vi "Marker Y Axes Values.vi"(0 "VISA resource name":refnum<visa-resource-name>, 5 "error in (no error)":errorcluster) -> (8 "o Marker A Value":dbl format="%^.3e", 9 "Right - Left Diff Curs Value":dbl format="%^.3e", 10 "x Marker A Value":dbl format="%^.3e", 11 "Line Curs Right Value":dbl format="%^.3e", 12 "o - x Diff Marker A Value":dbl format="%^.3e", 13 "Line Curs Left Value":dbl format="%^.3e", 14 "VISA resource name out":refnum<visa-resource-name>, 15 "o Marker B Value":dbl format="%^.3e", 16 "x Marker B Value":dbl format="%^.3e", 17 "o - x Diff Marker B Value":dbl format="%^.3e", 18 "Line Curs Value":dbl format="%^.3e", 19 "error out":errorcluster)   [LabVIEW 2017, in "Agilent 4194.lvlib"]
doc: "This function outputs the markers and cursors data valid for Y axis."
uses:
  ISOMems/Agilent 4194/Agilent 4194.lvlib
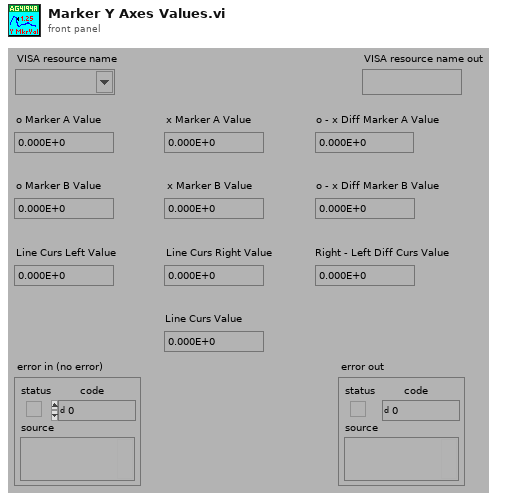
[diagram p1: front panel]
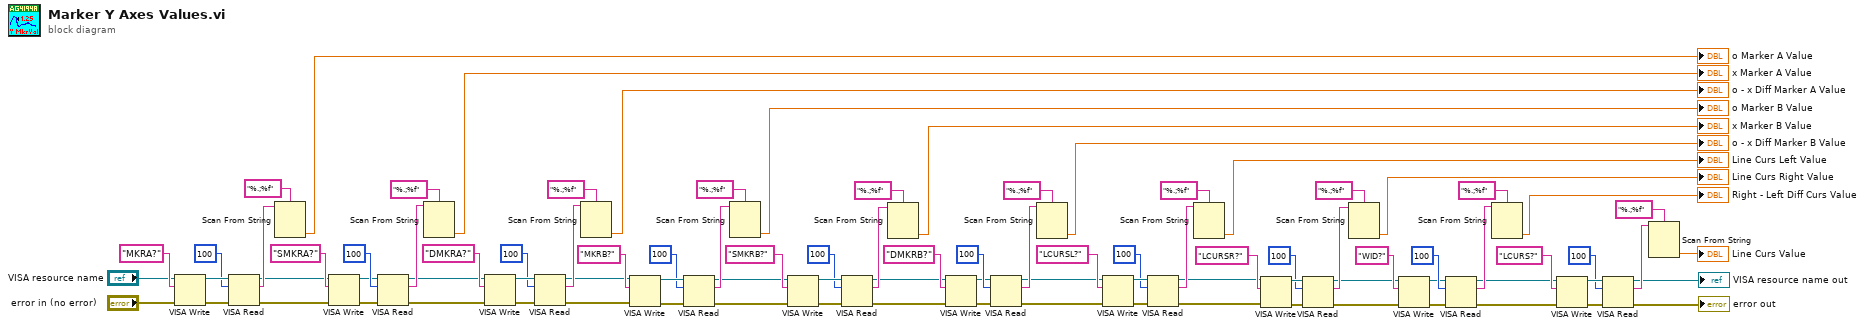
[diagram p0: block diagram]
diagram:
  n1 = VISA Write(VISA resource name="VISA resource name", write buffer="MKRA?" ("write buffer (\"\")"), error in (no error)="error in (no error)") -> (VISA resource name out=w32:refnum<visa-resource-name>, error out=w33:errorcluster)  [unwired: 1 out]
  n2 = VISA Read(VISA resource name=w32, byte count=u32 100 ("byte count (0)"), error in (no error)=w33) -> (VISA resource name out=w17:refnum<visa-resource-name>, read buffer=w29:string, error out=w16:errorcluster)  [unwired: 1 out]
  n3 = Scan From String(format string="%.;%f", input string=w29) -> (output 1=→"o Marker A Value":dbl)  [unwired: 3 in, 3 out]
  n4 = VISA Write(VISA resource name=w17, write buffer="SMKRA?" ("write buffer (\"\")"), error in (no error)=w16) -> (VISA resource name out=w25:refnum<visa-resource-name>, error out=w24:errorcluster)  [unwired: 1 out]
  n5 = VISA Read(VISA resource name=w25, byte count=u32 100 ("byte count (0)"), error in (no error)=w24) -> (VISA resource name out=w15:refnum<visa-resource-name>, read buffer=w27:string, error out=w14:errorcluster)  [unwired: 1 out]
  n6 = Scan From String(format string="%.;%f", input string=w27) -> (output 1=→"x Marker A Value":dbl)  [unwired: 3 in, 3 out]
  n7 = VISA Write(VISA resource name=w15, write buffer="DMKRA?" ("write buffer (\"\")"), error in (no error)=w14) -> (VISA resource name out=w22:refnum<visa-resource-name>, error out=w23:errorcluster)  [unwired: 1 out]
  n8 = VISA Read(VISA resource name=w22, byte count=u32 100 ("byte count (0)"), error in (no error)=w23) -> (VISA resource name out=w11:refnum<visa-resource-name>, read buffer=w20:string, error out=w10:errorcluster)  [unwired: 1 out]
  n9 = Scan From String(format string="%.;%f", input string=w20) -> (output 1=→"o - x Diff Marker A Value":dbl)  [unwired: 3 in, 3 out]
  n10 = VISA Write(VISA resource name=w11, write buffer="MKRB?" ("write buffer (\"\")"), error in (no error)=w10) -> (VISA resource name out=w37:refnum<visa-resource-name>, error out=w38:errorcluster)  [unwired: 1 out]
  n11 = VISA Read(VISA resource name=w37, byte count=u32 100 ("byte count (0)"), error in (no error)=w38) -> (VISA resource name out=w8:refnum<visa-resource-name>, read buffer=w34:string, error out=w9:errorcluster)  [unwired: 1 out]
  n12 = Scan From String(format string="%.;%f", input string=w34) -> (output 1=→"o Marker B Value":dbl)  [unwired: 3 in, 3 out]
  n13 = VISA Write(VISA resource name=w8, write buffer="SMKRB?" ("write buffer (\"\")"), error in (no error)=w9) -> (VISA resource name out=w69:refnum<visa-resource-name>, error out=w70:errorcluster)  [unwired: 1 out]
  n14 = VISA Read(VISA resource name=w69, byte count=u32 100 ("byte count (0)"), error in (no error)=w70) -> (VISA resource name out=w54:refnum<visa-resource-name>, read buffer=w66:string, error out=w53:errorcluster)  [unwired: 1 out]
  n15 = Scan From String(format string="%.;%f", input string=w66) -> (output 1=→"x Marker B Value":dbl)  [unwired: 3 in, 3 out]
  n16 = VISA Write(VISA resource name=w54, write buffer="DMKRB?" ("write buffer (\"\")"), error in (no error)=w53) -> (VISA resource name out=w62:refnum<visa-resource-name>, error out=w61:errorcluster)  [unwired: 1 out]
  n17 = VISA Read(VISA resource name=w62, byte count=u32 100 ("byte count (0)"), error in (no error)=w61) -> (VISA resource name out=w52:refnum<visa-resource-name>, read buffer=w64:string, error out=w51:errorcluster)  [unwired: 1 out]
  n18 = Scan From String(format string="%.;%f", input string=w64) -> (output 1=→"o - x Diff Marker B Value":dbl)  [unwired: 3 in, 3 out]
  n19 = VISA Write(VISA resource name=w52, write buffer="LCURSL?" ("write buffer (\"\")"), error in (no error)=w51) -> (VISA resource name out=w59:refnum<visa-resource-name>, error out=w60:errorcluster)  [unwired: 1 out]
  n20 = VISA Read(VISA resource name=w59, byte count=u32 100 ("byte count (0)"), error in (no error)=w60) -> (VISA resource name out=w48:refnum<visa-resource-name>, read buffer=w57:string, error out=w47:errorcluster)  [unwired: 1 out]
  n21 = Scan From String(format string="%.;%f", input string=w57) -> (output 1=→"Line Curs Left Value":dbl)  [unwired: 3 in, 3 out]
  n22 = VISA Write(VISA resource name=w48, write buffer="LCURSR?" ("write buffer (\"\")"), error in (no error)=w47) -> (VISA resource name out=w91:refnum<visa-resource-name>, error out=w92:errorcluster)  [unwired: 1 out]
  n23 = VISA Read(VISA resource name=w91, byte count=u32 100 ("byte count (0)"), error in (no error)=w92) -> (VISA resource name out=w76:refnum<visa-resource-name>, read buffer=w88:string, error out=w75:errorcluster)  [unwired: 1 out]
  n24 = Scan From String(format string="%.;%f", input string=w88) -> (output 1=→"Line Curs Right Value":dbl)  [unwired: 3 in, 3 out]
  n25 = VISA Write(VISA resource name=w76, write buffer="WID?" ("write buffer (\"\")"), error in (no error)=w75) -> (VISA resource name out=w84:refnum<visa-resource-name>, error out=w83:errorcluster)  [unwired: 1 out]
  n26 = VISA Read(VISA resource name=w84, byte count=u32 100 ("byte count (0)"), error in (no error)=w83) -> (VISA resource name out=w74:refnum<visa-resource-name>, read buffer=w86:string, error out=w73:errorcluster)  [unwired: 1 out]
  n27 = Scan From String(format string="%.;%f", input string=w86) -> (output 1=→"Right - Left Diff Curs Value":dbl)  [unwired: 3 in, 3 out]
  n28 = VISA Write(VISA resource name=w74, write buffer="LCURS?" ("write buffer (\"\")"), error in (no error)=w73) -> (VISA resource name out=w81:refnum<visa-resource-name>, error out=w82:errorcluster)  [unwired: 1 out]
  n29 = VISA Read(VISA resource name=w81, byte count=u32 100 ("byte count (0)"), error in (no error)=w82) -> (VISA resource name out=→"VISA resource name out":refnum<visa-resource-name>, read buffer=w79:string, error out=→"error out":errorcluster)  [unwired: 1 out]
  n30 = Scan From String(format string="%.;%f", input string=w79) -> (output 1=→"Line Curs Value":dbl)  [unwired: 3 in, 3 out]
